vi "Output Item Init Common.vi"(8 "error in (no error)":errorcluster, 9 "UI Elements":T1, 10 "Output":T2, 11 "VI in":refnum<vi>) -> (0 "error out":errorcluster)   [LabVIEW 2015, in "OutputUI.lvclass"]
uses:
  OutputUI.lvclass
  Step/STEP_OUTPUT.ctl
  Step/OUTPUT_DATA_TYPE.ctl
  OUTPUT_CHECK_TYPE.ctl
  Step/OUTPUT_VALUE_TYPE.ctl
  <vilib>/Utility/miscctls.llb/LVPointTypeDef.ctl
  Step.lvclass
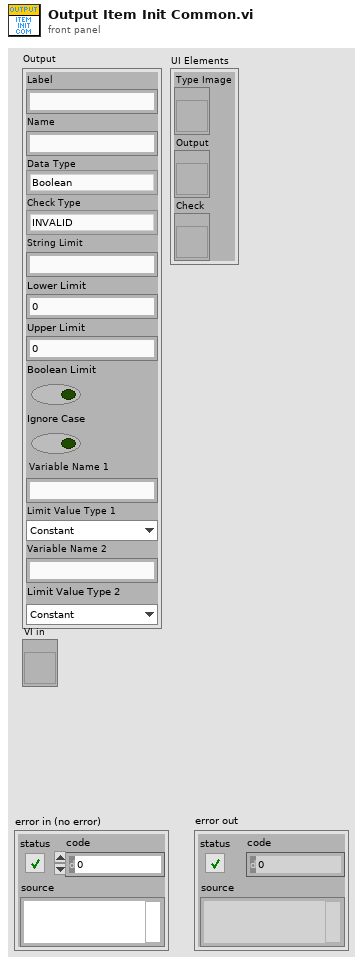
[diagram p1: front panel]
types:
  T1 = cluster{"Type Image":refnum<vi>, "Output":refnum<vi>, "Check":refnum<vi>}
  T2 = typedef "Step.lvclass/STEP_OUTPUT.ctl" = cluster{"Label":string, "Name":string, "Data Type":T3, "Check Type":T4, "String Limit":string, "Lower Limit":dbl, "Upper Limit":dbl, "Boolean Limit":bool, "Ignore Case":bool, "Variable Name 1":string, "Limit Value Type 1":T5, "Variable Name 2":string, "Limit Value Type 2":T5}
  T3 = typedef "Step.lvclass/OUTPUT_DATA_TYPE.ctl" = enum16{"Boolean", "String", "Numeric", "Other"}
  T4 = typedef "Step.lvclass/OUTPUT_CHECK_TYPE.ctl" = enum16{"INVALID", "DO_NOT_CHECK", "RECORD", "VARIABLE", "EQUAL", "NOT_EQUAL", "STR_CONTAINS", "STR_START_WITH", "STR_END_WITH", "STR_REGEX_MATCH", "NUM_GT", "NUM_LT", "NUM_GE", "NUM_LE", "NUM_RANGE", "NUM_RANGE_BDY"}
  T5 = typedef "Step.lvclass/OUTPUT_VALUE_TYPE.ctl" = enum16{"Constant", "Variable"}
  T6 = typedef "LVPointTypeDef.ctl" = cluster{"Horizontal":i16, "Vertical":i16}
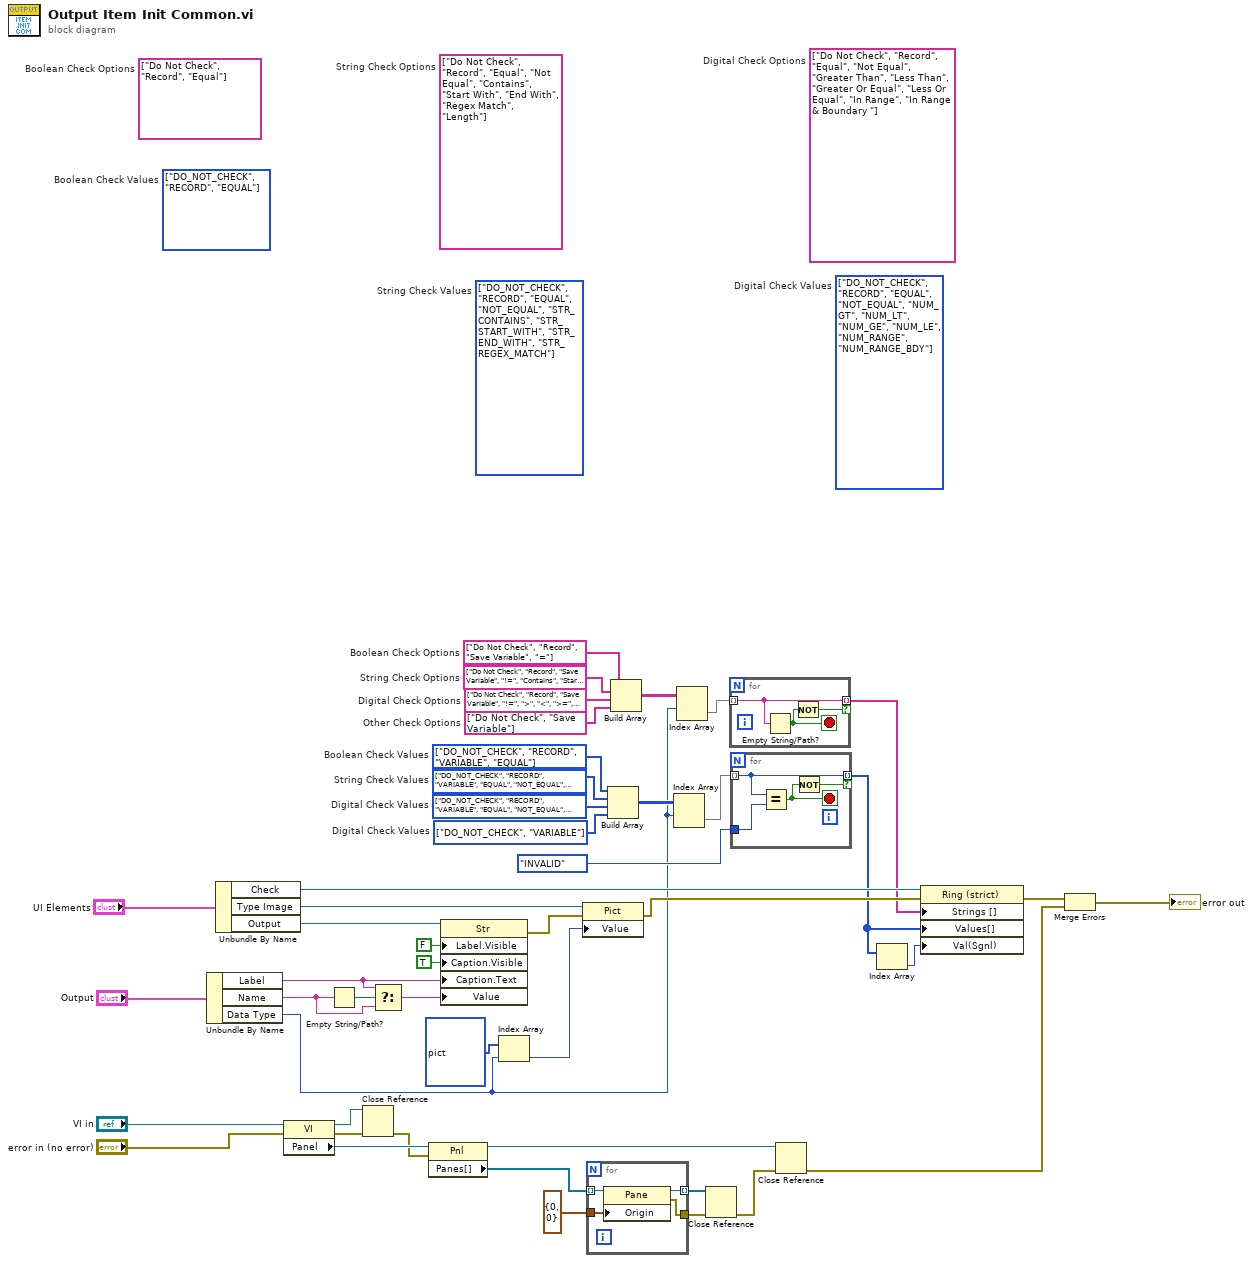
[diagram p0: block diagram]
diagram:
  w3 = T4[] [enum."DO_NOT_CHECK", enum."VARIABLE"] items=["INVALID", "DO_NOT_CHECK", "RECORD", "VARIABLE", "EQUAL", "NOT_EQUAL", "STR_CONTAINS", "STR_START_WITH", "STR_END_WITH", "STR_REGEX_MATCH", "NUM_GT", "NUM_LT", "NUM_GE", "NUM_LE", "NUM_RANGE", "NUM_RANGE_BDY"]  # Digital Check Values
  w4 = string[] ["Do Not Check", "Save Variable"]  # Other Check Options
  w10 = T4[] [enum."DO_NOT_CHECK", enum."RECORD", enum."VARIABLE", enum."EQUAL", enum."NOT_EQUAL", enum."NUM_GT", enum."NUM_LT", enum."NUM_GE", enum."NUM_LE", enum."NUM_RANGE", enum."NUM_RANGE_BDY"] items=["INVALID", "DO_NOT_CHECK", "RECORD", "VARIABLE", "EQUAL", "NOT_EQUAL", "STR_CONTAINS", "STR_START_WITH", "STR_END_WITH", "STR_REGEX_MATCH", "NUM_GT", "NUM_LT", "NUM_GE", "NUM_LE", "NUM_RANGE", "NUM_RANGE_BDY"]  # Digital Check Values
  w11 = T4[] [enum."DO_NOT_CHECK", enum."RECORD", enum."VARIABLE", enum."EQUAL", enum."NOT_EQUAL", enum."STR_CONTAINS", enum."STR_START_WITH", enum."STR_END_WITH", enum."STR_REGEX_MATCH"] items=["INVALID", "DO_NOT_CHECK", "RECORD", "VARIABLE", "EQUAL", "NOT_EQUAL", "STR_CONTAINS", "STR_START_WITH", "STR_END_WITH", "STR_REGEX_MATCH", "NUM_GT", "NUM_LT", "NUM_GE", "NUM_LE", "NUM_RANGE", "NUM_RANGE_BDY"]  # String Check Values
  w12 = T4[] [enum."DO_NOT_CHECK", enum."RECORD", enum."VARIABLE", enum."EQUAL"] items=["INVALID", "DO_NOT_CHECK", "RECORD", "VARIABLE", "EQUAL", "NOT_EQUAL", "STR_CONTAINS", "STR_START_WITH", "STR_END_WITH", "STR_REGEX_MATCH", "NUM_GT", "NUM_LT", "NUM_GE", "NUM_LE", "NUM_RANGE", "NUM_RANGE_BDY"]  # Boolean Check Values
  (unwired) T4[] [enum."DO_NOT_CHECK", enum."RECORD", enum."EQUAL", enum."NOT_EQUAL", enum."NUM_GT", enum."NUM_LT", enum."NUM_GE", enum."NUM_LE", enum."NUM_RANGE", enum."NUM_RANGE_BDY"] items=["INVALID", "DO_NOT_CHECK", "RECORD", "VARIABLE", "EQUAL", "NOT_EQUAL", "STR_CONTAINS", "STR_START_WITH", "STR_END_WITH", "STR_REGEX_MATCH", "NUM_GT", "NUM_LT", "NUM_GE", "NUM_LE", "NUM_RANGE", "NUM_RANGE_BDY"]  # Digital Check Values
  (unwired) T4[] [enum."DO_NOT_CHECK", enum."RECORD", enum."EQUAL", enum."NOT_EQUAL", enum."STR_CONTAINS", enum."STR_START_WITH", enum."STR_END_WITH", enum."STR_REGEX_MATCH"] items=["INVALID", "DO_NOT_CHECK", "RECORD", "VARIABLE", "EQUAL", "NOT_EQUAL", "STR_CONTAINS", "STR_START_WITH", "STR_END_WITH", "STR_REGEX_MATCH", "NUM_GT", "NUM_LT", "NUM_GE", "NUM_LE", "NUM_RANGE", "NUM_RANGE_BDY"]  # String Check Values
  (unwired) T4[] [enum."DO_NOT_CHECK", enum."RECORD", enum."EQUAL"] items=["INVALID", "DO_NOT_CHECK", "RECORD", "VARIABLE", "EQUAL", "NOT_EQUAL", "STR_CONTAINS", "STR_START_WITH", "STR_END_WITH", "STR_REGEX_MATCH", "NUM_GT", "NUM_LT", "NUM_GE", "NUM_LE", "NUM_RANGE", "NUM_RANGE_BDY"]  # Boolean Check Values
  (unwired) string[] ["Do Not Check", "Record", "Equal"]  # Boolean Check Options
  (unwired) string[] ["Do Not Check", "Record", "Equal", "Not Equal", "Contains", "Start With", "End With", "Regex Match", "Length"]  # String Check Options
  w19 = string[] ["Do Not Check", "Record", "Save Variable", "=", "!=", "Contains", "Start With", "End With", "Regex Match"]  # String Check Options
  (unwired) string[] ["Do Not Check", "Record", "Equal", "Not Equal", "Greater Than", "Less Than", "Greater Or Equal", "Less Or Equal", "In Range", "In Range & Boundary "]  # Digital Check Options
  w20 = string[] ["Do Not Check", "Record", "Save Variable", "=", "!=", ">", "<", ">=", "<=", "> & <", ">= & <="]  # Digital Check Options
  w22 = string[] ["Do Not Check", "Record", "Save Variable", "="]  # Boolean Check Options
  n1 = Unbundle By Name("Output") -> ("Label"=w31:string, "Name"=w30:string, "Data Type"=w8:T3)
  n2 = Unbundle By Name("UI Elements") -> ("Check"=w24:refnum<vi>, "Type Image"=w28:refnum<vi>, "Output"=w35:refnum<vi>)
  n3 = property class="VI"(reference="VI in", error in="error in (no error)") -> (reference out=w39:refnum<vi>, error out=w40:errorcluster, "Panel"=w42:refnum<vi>)
  n4 = Empty String/Path?(string/path=w30) -> (empty?=w32:bool)
  n5 = Close Reference(reference=w39, error in (no error)=w40) -> (error out=w38:errorcluster)
  n6 = Select(t=w31, s=w32, f=w30) -> (s? t:f=w29:string)
  n7 = property class="Pnl"(reference=w42, error in=w38) -> (reference out=w37:refnum<vi>, "Panes[]"=w44:refnum<vi>[])  [unwired: 1 out]
  n8 = property class="Str"(reference=w35, "Label.Visible"=FALSE, "Caption.Visible"=TRUE, "Caption.Text"=w31, "Value"=w29) -> (error out=w25:errorcluster)  [unwired: 1 in, 1 out]
  n9 = Index Array(array=picture[] [bytes[530], bytes[530], bytes[510], bytes[275]], index=w8) -> (element=w26:picture)
  n10 = property class="Pict"(reference=w28, error in=w25, "Value"=w26) -> (error out=w23:errorcluster)  [unwired: 1 out]
  n11 = for {
    tunnel: w44 -> [w51] mode=indexing
    tunnel: T6 {"Horizontal"=0, "Vertical"=0} ("Origin") -> [w50]
    tunnel: [w49] -> w46 mode=indexing
    tunnel: [w48] -> w47
    n12 = property class="Pane"(reference=w51, "Origin"=w50) -> (reference out=w49:refnum<vi>, error out=w48:errorcluster)  [unwired: 1 in]
  }
  n13 = Build Array(w12, w11, w10, w3) -> (w13:T4[][])
  n14 = Build Array(w22, w19, w20, w4) -> (w21:string[][])
  n15 = Index Array(array=w13, index (row)=w8) -> (element=w14:T4[])  [unwired: 1 in]
  n16 = Index Array(array=w21, index (row)=w8) -> (element=w18:string[])  [unwired: 1 in]
  n17 = Close Reference(reference=w46, error in (no error)=w47) -> (error out=w36:errorcluster)
  n18 = for {
    tunnel: w18 -> [w54] mode=indexing
    tunnel: [w54] -> w17 mode=indexing if=w53
    stop <- w52 stop-if-true
    n19 = Empty String/Path?(string/path=w54) -> (empty?=w52:bool)
    n20 = Not(x=w52) -> (.not. x?=w53:bool)
  }
  n21 = for {
    tunnel: w14 -> [w56] mode=indexing
    tunnel: [w56] -> w7 mode=indexing if=w58
    tunnel: OUTPUT_CHECK_TYPE."INVALID" ("Check Type") -> [w55]
    stop <- w57 stop-if-true
    n22 = Equal?(x=w56, y=w55) -> (x = y?=w57:bool)
    n23 = Not(x=w57) -> (.not. x?=w58:bool)
  }
  n24 = Close Reference(reference=w37, error in (no error)=w36) -> (error out=w15:errorcluster)
  n25 = Index Array(array=w7) -> (element=w6:T4)  [unwired: 1 in]
  n26 = property class="Ring (strict)"(reference=w24, error in=w23, "Strings []"=w17, "Values[]"=w7, "Val(Sgnl)"=w6) -> (error out=w16:errorcluster)  [unwired: 1 out]
  n27 = Merge Errors(w16, w15) -> (→"error out":errorcluster)
